vi "Reset Host Buffer I64.vi"(7 "index":i32, 8 "error in":errorcluster, 11 "fpga session in":refnum<k20>) -> (0 "error out":errorcluster, 3 "fpga session out":refnum<k20>)   [LabVIEW 2018, in "Lock-In Amplifier Example Host.lvlib"]
uses:
  Lock-In Amplifier Example Host.lvlib
  fpga type.ctl
  <vilib>/Utility/error.llb/Error Cluster From Error Code.vi
  <vilib>/rvi/interface/nirviMethod/nirviMethod.xnode
  <vilib>/ErrorRing/Error Ring.xnode
  <vilib>/FPGAPlugInAG/Dynamic/niLvFpga_StopFifo_Dynamic.vi
  <vilib>/rvi/errors/niLvFpgaMergeErrorWithErrorCode.vi
  <vilib>/FPGAPlugInAG/Dynamic/niLvFpga_StartFifo_Dynamic.vi
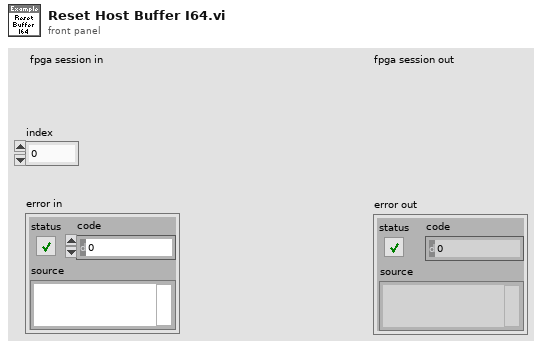
[diagram p1: front panel]
types:
  T1 = typedef "Lock-In Amplifier Example Host.lvlib/fpga type.ctl" = refnum<k20>
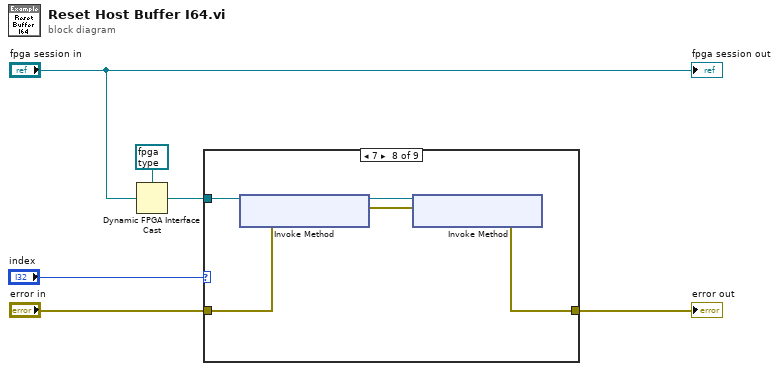
[diagram p0: block diagram]
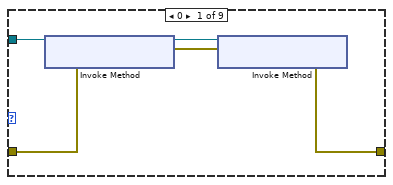
[diagram p2: hidden frame]
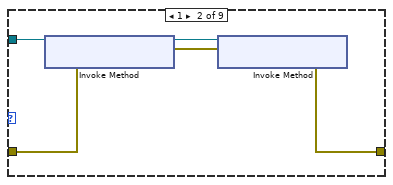
[diagram p3: hidden frame]
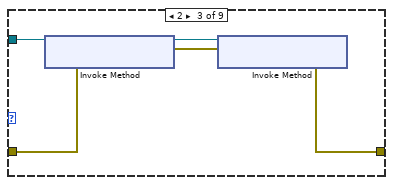
[diagram p4: hidden frame]
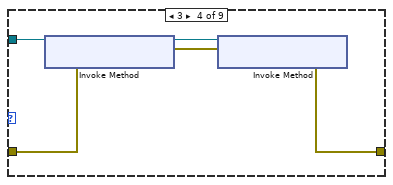
[diagram p5: hidden frame]
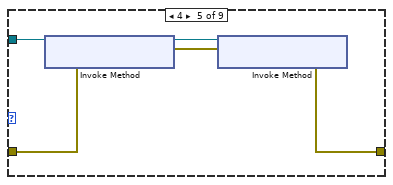
[diagram p6: hidden frame]
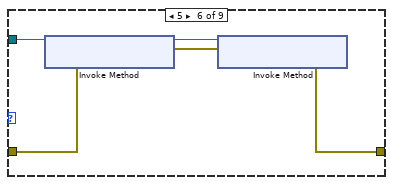
[diagram p7: hidden frame]
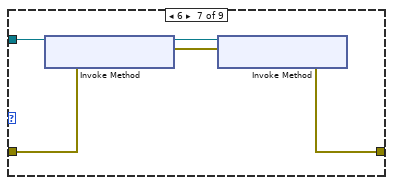
[diagram p8: hidden frame]
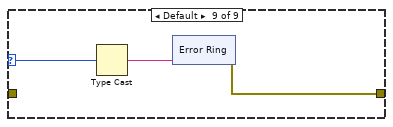
[diagram p9: hidden frame]
diagram:
  n1 = Dynamic FPGA Interface Cast(Session In=T1 refnum ("fpga type"), Type="fpga session in") -> (Session Out=w4:T1)
  n2 = case shown="7" "index" {
    selector: "index" -> [_ _ _ _ _ _ _ _ w48]
    tunnel: w4 -> [w11 w16 w21 w26 w31 w36 w41 w46 _]
    tunnel: "error in" -> [w8 w13 w18 w23 w28 w33 w38 w43 _]
    tunnel: [w7 w12 w17 w22 w27 w32 w37 w42 w49] -> w2
    frame 0 {
      n3 = xnode "Invoke Method"("FPGA VI Reference In"=w11, "error in"=w8) -> ("FPGA VI Reference Out"=w9:T1, "error out"=w10:errorcluster)
      n4 = xnode "Invoke Method"("FPGA VI Reference In"=w9, "error in"=w10) -> ("error out"=w7:errorcluster)  [unwired: 1 out]
    }
    frame 1 {
      n5 = xnode "Invoke Method"("FPGA VI Reference In"=w16, "error in"=w13) -> ("FPGA VI Reference Out"=w14:T1, "error out"=w15:errorcluster)
      n6 = xnode "Invoke Method"("FPGA VI Reference In"=w14, "error in"=w15) -> ("error out"=w12:errorcluster)  [unwired: 1 out]
    }
    frame 2 {
      n7 = xnode "Invoke Method"("FPGA VI Reference In"=w21, "error in"=w18) -> ("FPGA VI Reference Out"=w19:T1, "error out"=w20:errorcluster)
      n8 = xnode "Invoke Method"("FPGA VI Reference In"=w19, "error in"=w20) -> ("error out"=w17:errorcluster)  [unwired: 1 out]
    }
    frame 3 {
      n9 = xnode "Invoke Method"("FPGA VI Reference In"=w26, "error in"=w23) -> ("FPGA VI Reference Out"=w24:T1, "error out"=w25:errorcluster)
      n10 = xnode "Invoke Method"("FPGA VI Reference In"=w24, "error in"=w25) -> ("error out"=w22:errorcluster)  [unwired: 1 out]
    }
    frame 4 {
      n11 = xnode "Invoke Method"("FPGA VI Reference In"=w31, "error in"=w28) -> ("FPGA VI Reference Out"=w29:T1, "error out"=w30:errorcluster)
      n12 = xnode "Invoke Method"("FPGA VI Reference In"=w29, "error in"=w30) -> ("error out"=w27:errorcluster)  [unwired: 1 out]
    }
    frame 5 {
      n13 = xnode "Invoke Method"("FPGA VI Reference In"=w36, "error in"=w33) -> ("FPGA VI Reference Out"=w34:T1, "error out"=w35:errorcluster)
      n14 = xnode "Invoke Method"("FPGA VI Reference In"=w34, "error in"=w35) -> ("error out"=w32:errorcluster)  [unwired: 1 out]
    }
    frame 6 {
      n15 = xnode "Invoke Method"("FPGA VI Reference In"=w41, "error in"=w38) -> ("FPGA VI Reference Out"=w39:T1, "error out"=w40:errorcluster)
      n16 = xnode "Invoke Method"("FPGA VI Reference In"=w39, "error in"=w40) -> ("error out"=w37:errorcluster)  [unwired: 1 out]
    }
    frame 7 {
      n17 = xnode "Invoke Method"("FPGA VI Reference In"=w46, "error in"=w43) -> ("FPGA VI Reference Out"=w44:T1, "error out"=w45:errorcluster)
      n18 = xnode "Invoke Method"("FPGA VI Reference In"=w44, "error in"=w45) -> ("error out"=w42:errorcluster)  [unwired: 1 out]
    }
    frame Default {
      n19 = Type Cast(x=w48) -> (*(type *) &x=w47:string)  [unwired: 1 in]
      n20 = xnode "Error Ring"("parameter 0"=w47) -> ("error out"=w49:errorcluster)
    }
  }
  "error out" <- w2
  "fpga session out" <- "fpga session in"
